vi "Main-Auto.vi"() -> ()   [LabVIEW 2019]
uses:
  <vilib>/Platform/TimedLoop/XDataNode/timing_clust.ctl
  <vilib>/Platform/TimedLoop/XDataNode/nitl_modes.ctl
  <vilib>/Platform/TimedLoop/XDataNode/wakeup.ctl
  <vilib>/myRIO/Instrument Drivers/Onboard IO/DIO/typedefs/DIO Reference.ctl
  <vilib>/myRIO/Common/Instrument Driver Framework/Utilities/typedefs/myRIO Generic Hardware Reference.ctl
  <vilib>/myRIO/Common/Instrument Driver Framework/Utilities/typedefs/Hardware Version Enum.ctl
  <vilib>/myRIO/Common/Instrument Driver Framework/Utilities/typedefs/myRIO v1.0 Reference.ctl
  <vilib>/myRIO/Common/Instrument Driver Framework/Utilities/typedefs/Generic FPGA Reference.ctl
  <vilib>/myRIO/Common/Instrument Driver Framework/myRIO v1.0/DIO/typedefs/DIO Channels List.ctl
  <vilib>/myRIO/Common/Instrument Driver Framework/myRIO v1.0/DIO/typedefs/DIO Channels Enum.ctl
  <vilib>/userDefined/High Color/nirio_resource_hc.ctl
  <vilib>/myRIO/Common/Instrument Driver Framework/Utilities/vis/Is FPGA Ref Available.vi
  <vilib>/myRIO/Common/Instrument Driver Framework/myRIO v1.0/DIO/vis/myRIO v1.1 Open DIO.vi
  <vilib>/myRIO/Instrument Drivers/Onboard IO/DIO/vis/Write.vi
  <vilib>/myRIO/Common/Instrument Driver Framework/Utilities/vis/Validate Channels.vi
  <vilib>/myRIO/Common/Instrument Driver Framework/myRIO v1.0/DIO/vis/myRIO v1.0 Reserve DIO.vi
  <vilib>/myRIO/Common/Instrument Driver Framework/myRIO v1.0/UART/vis/myRIO v1.0 Close UART.vi
  <vilib>/myRIO/Common/Instrument Driver Framework/myRIO v1.0/Resource Manager/vis/myRIO v1.0 Reserve Channel List.vi
  <vilib>/myRIO/Common/Instrument Driver Framework/myRIO v1.0/DIO/vis/myRIO v1.0 Build MUX Configuration DIO.vi
  <vilib>/myRIO/Common/Instrument Driver Framework/myRIO v1.0/Resource Manager/vis/myRIO v1.0 Reserve Channel.vi
  <vilib>/myRIO/Common/Instrument Driver Framework/myRIO v1.0/Resource Manager/vis/myRIO v1.0 Unreserve Channel.vi
  <vilib>/myRIO/Common/Instrument Driver Framework/myRIO v1.0/Resource Manager/vis/myRIO v1.0 Create Configuration List.vi
  <vilib>/myRIO/Common/Instrument Driver Framework/myRIO v1.0/Resource Manager/vis/myRIO v1.0 Build Mutex Name.vi
  Sub VI/Variable/Lock-PID.vi
  <vilib>/Utility/VariantDataType/GetNumericInfo.vi
  <vilib>/Utility/error.llb/Error Cluster From Error Code.vi
  <vilib>/myRIO/Common/Instrument Driver Framework/myRIO v1.0/myRIO v1.1 Open.vi
  <vilib>/myRIO/Common/Instrument Driver Framework/Utilities/vis/IO Manager.vi
  <vilib>/myRIO/Common/Instrument Driver Framework/Utilities/vis/Configuration Manager.vi
  <vilib>/myRIO/Common/Instrument Driver Framework/myRIO v1.0/Resource Manager/vis/myRIO v1.0 Configure IO.vi
  <vilib>/myRIO/Common/Instrument Driver Framework/myRIO v1.0/myRIO v1.0 Close.vi
  <vilib>/myRIO/Common/Instrument Driver Framework/myRIO v1.0/DIO/vis/myRIO v1.0 Write DIO.vi
  Sub VI/Variable/Go-Home.vi
  <vilib>/myRIO/Common/Instrument Driver Framework/Utilities/vis/FPGA Ref Manager.vi
  <vilib>/myRIO/Common/Instrument Driver Framework/myRIO v1.0/myRIO v1.0 Reset FPGA.vi
  <vilib>/myRIO/Common/Instrument Driver Framework/myRIO v1.0/IRQ/vis/myRIO v1.0 IRQ Info FGV.vi
  <vilib>/myRIO/Common/Instrument Driver Framework/myRIO v1.0/IRQ/vis/myRIO v1.0 Timer IRQ Info FGV.vi
  <vilib>/myRIO/Common/Instrument Driver Framework/myRIO v1.0/IRQ/vis/myRIO v1.0 ISR Agent.vi
  <vilib>/myRIO/Instrument Drivers/Utilities/vis/Reset Index.vi
  <vilib>/myRIO/Common/Instrument Driver Framework/myRIO v1.0/Resource Manager/vis/myRIO v1.0 Block Write Resource Manager.vi
  <vilib>/platform/TimedLoop/XDataNode/XDataNode.xnode
  <vilib>/myRIO/Express VI/Onboard Devices/LED/LED Express VI.xnode
  <vilib>/myRIO/Instrument Drivers/Onboard IO/DIO/vis/myRIO DIO Open.xnode
  <vilib>/myRIO/Instrument Drivers/Utilities/Utilities.lvlib
  <vilib>/Platform/TimedLoop/XDataNode/XDNodeRunTimeDep.lvlib
  <vilib>/myRIO/Instrument Drivers/Onboard IO/DIO/DIO.lvlib
panel:
  out "總辨識機率":i32[](graph)
  out "第二次辨識機率":i32[](graph)
  out "第一次辨識機率":i32[](graph)
  out "辨識機率":dbl[](array[slide]) scale=0.0..10.0
  out "總辨識結果":string[](array[string])
  out "輸出顏色-位置":T1(array[cluster])
  out "當前動作":enum16{"辨識", "夾球+回橋"}(ring)
  in  "Stop":bool
  out "Error Out":errorcluster
  in  "Error In":errorcluster
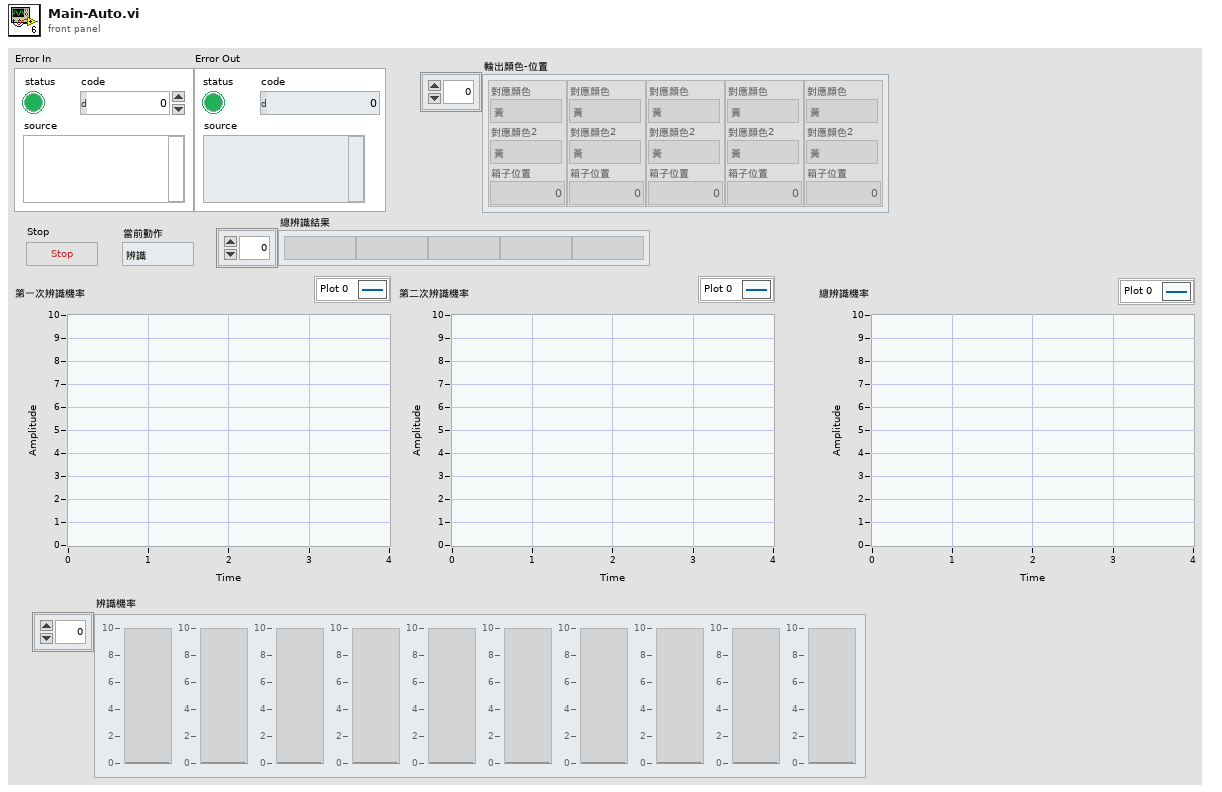
[diagram p1: front panel]
types:
  T1 = cluster{"對應顏色":enum16{"黃", "紅", "綠", "藍", "黑", "無"}, "對應顏色2":enum16{"黃", "紅", "綠", "藍", "黑", "無"}, "箱子位置":i32}[]
  T2 = enum16{"第一次夾球", "第二次夾球", "第三次夾球", "第四次夾球", "第五次夾球"}
  T3 = enum16{"第一次夾球", "第二次夾球", "第三次夾球", "第四次夾球", "第五次夾球"}[]
  T4 = typedef "I2C.lvlib/I2C Reference.ctl" = cluster{"myRIO Reference":T5, "I2C Channels Enum":T9, "I2C Configuration":T10}
  T5 = typedef "myRIO Generic Hardware Reference.ctl" = cluster{"myRIO Model":T6, "myRIO Hardware Reference":T7}
  T6 = typedef "Hardware Version Enum.ctl" = enum16{"Unknown", "myRIO-1900", "myRIO-1950", "roboRIO", "NI ELVIS RIO CM", "ELVIS III"}
  T7 = typedef "myRIO v1.0 Reference.ctl" = cluster{"Generic FPGA Reference":T8, "Allow multiple opens":bool}
  T8 = typedef "Generic FPGA Reference.ctl" = refnum<k20>
  T9 = typedef "I2C Channels Enum.ctl" = enum16{"Not Connected", "A/I2C", "B/I2C", "I2C/I2C"}
  T10 = typedef "I2C.lvlib/I2C Configuration.ctl" = cluster{"I2C Transfer Rate":T11}
  T11 = typedef "I2C.lvlib/I2C Transfer Rate.ctl" = enum16{"Standard mode (100 kbps)", "Fast mode (400 kbps)"}
  T12 = cluster{"Array":i32[], "Array":i32[], "Array":i32[]}
  T13 = typedef "XDNodeRunTimeDep.lvlib/timing_clust.ctl" = cluster{"Expected End [f-1]":u64, "Actual End [f-1]":u64, "Finished Late? [f-1]":bool, "Expected End [i-1]":u64, "Actual End [i-1]":u64, "Finished Late? [i-1]":bool, "Expected Start [i]":u64, "Actual Start [i]":u64, "Expected Start [f]":u64, "Actual Start [f]":u64, "Source Name":string, "Structure Name":string, "Period":i64, "Deadline":i64, "Offset":i64, "Start":i64, "Priority":i32, "Timeout":i32, "Mode":T14, "Wakeup Reason":T15, "Error":errorcluster, "Source Type":string, "Secondary Source Type":string, "Global End Time":u64, "Global Start Time":u64, "Frame Duration":u64, "Iteration Duration":u64, "Assigned CPU":i32, "I/O Scan Engine Mode":u32}
  T14 = typedef "XDNodeRunTimeDep.lvlib/nitl_modes.ctl" = enum32{"No Change", "Process missed periods, maintain original phase", "Discard missed periods, maintain original phase", "Process missed periods, ignore original phase", "Discard missed periods, ignore original phase"}
  T15 = typedef "XDNodeRunTimeDep.lvlib/wakeup.ctl" = enum32{"Normal", "Aborted", "Asynchronous wakeup", "Timing source error", "Timed loop error", "Timeout"}
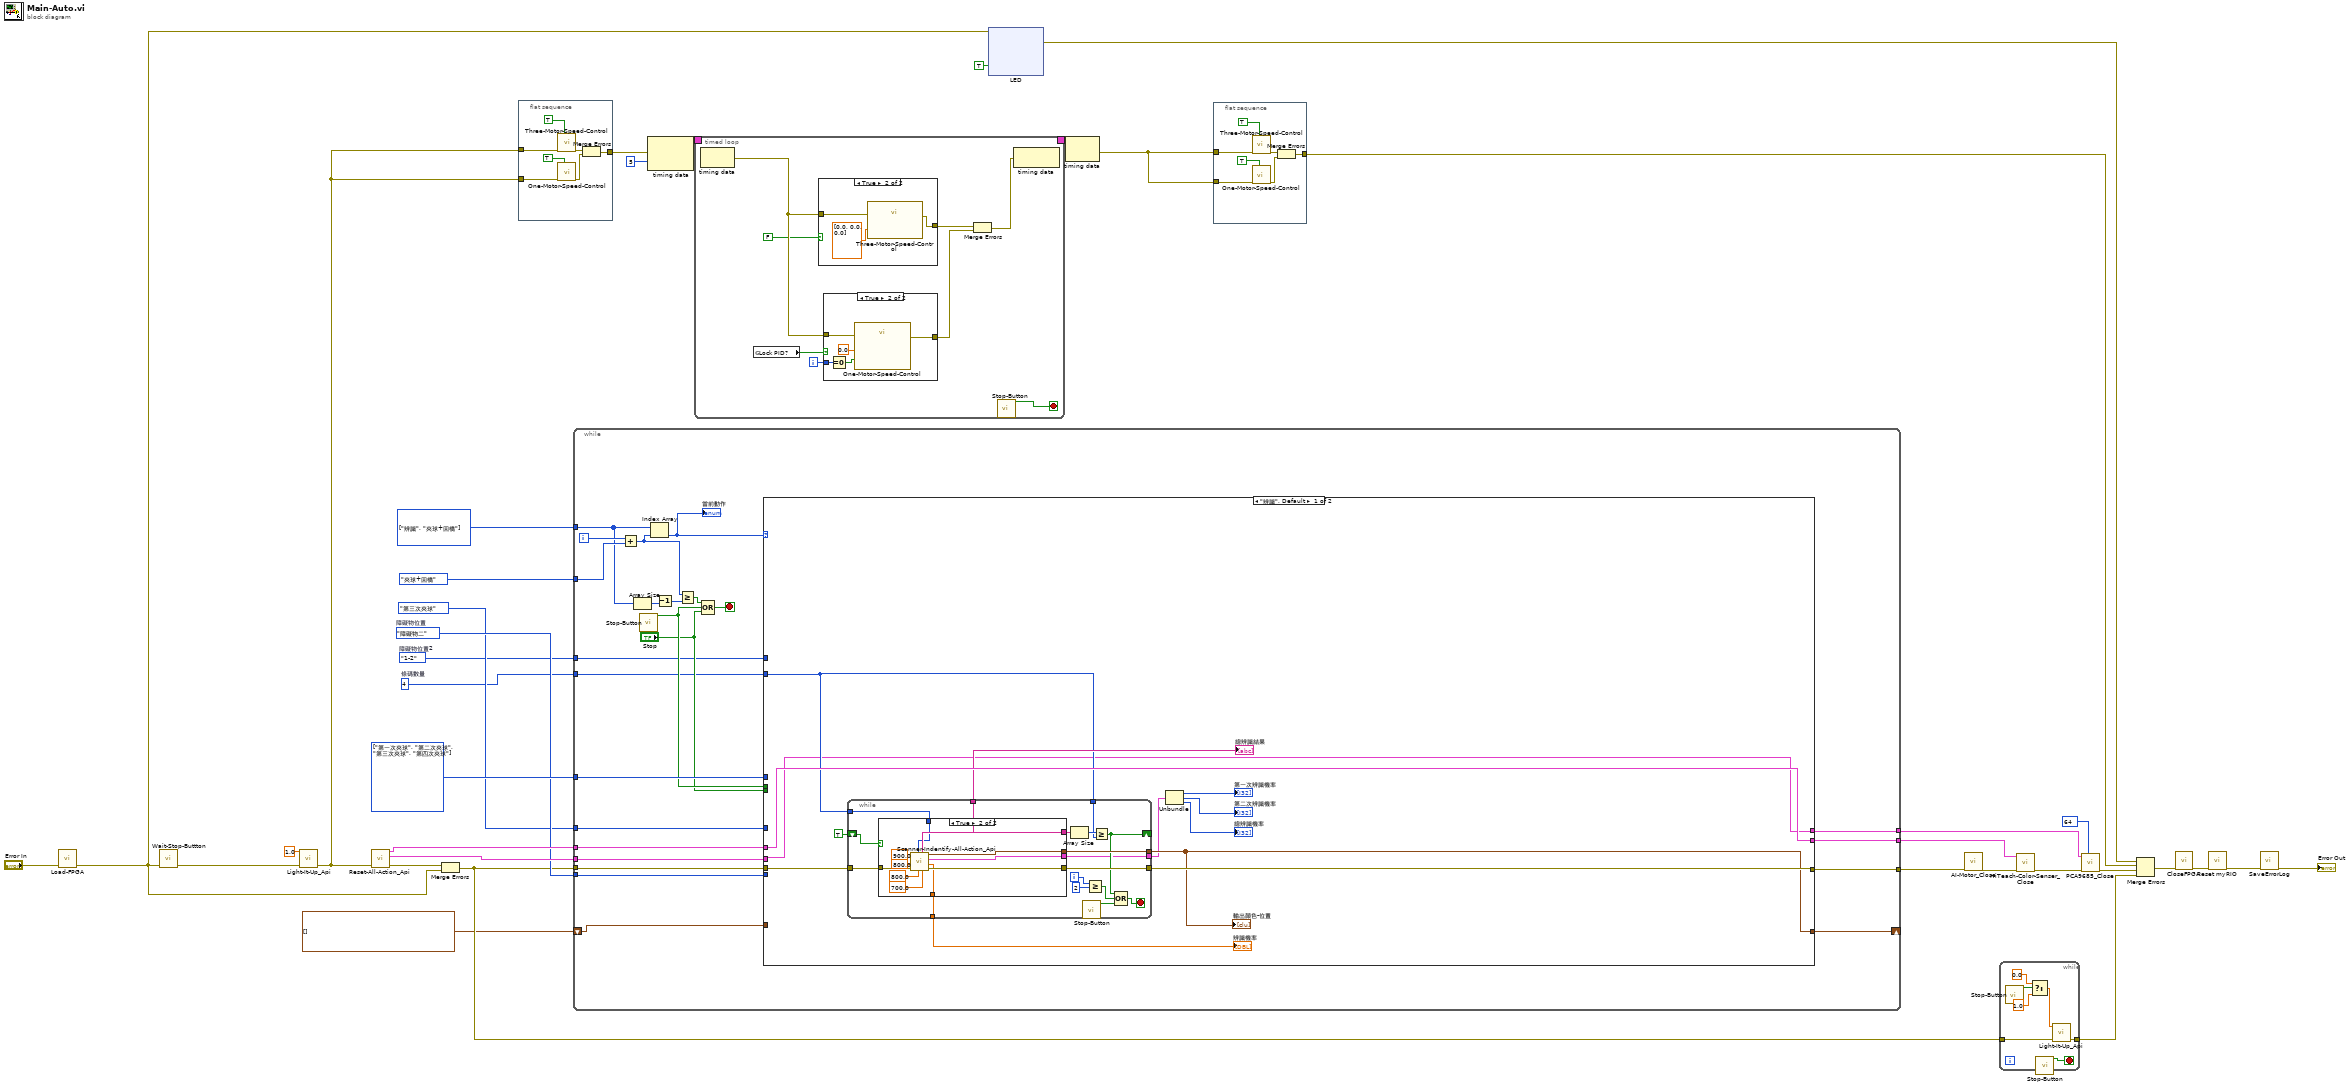
[diagram p0: block diagram]
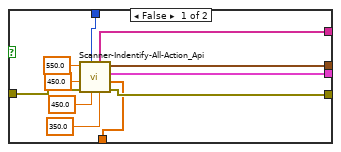
[diagram p2: hidden frame]
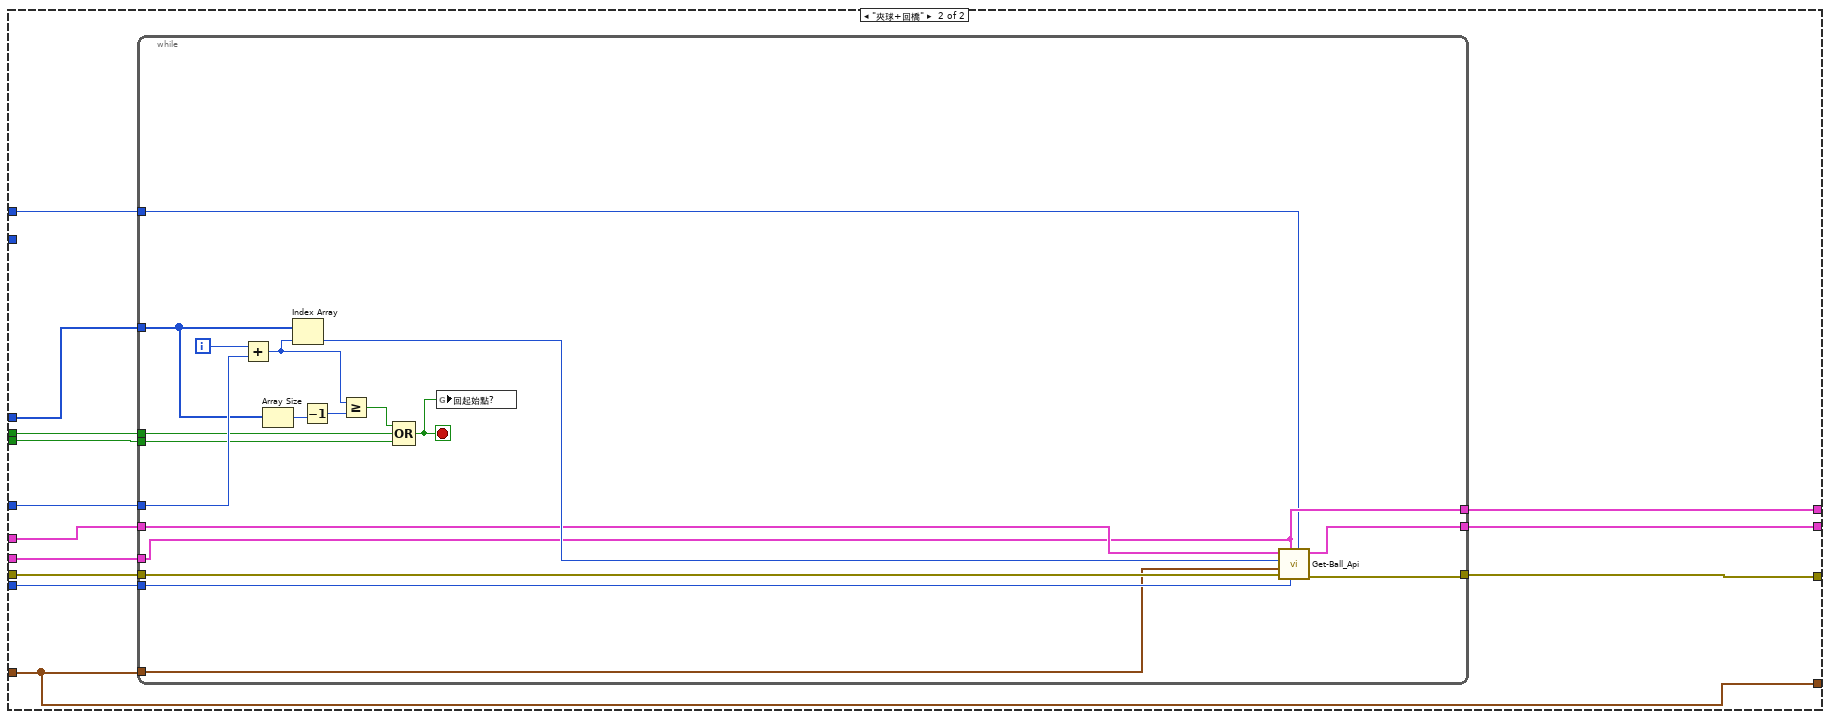
[diagram p3: hidden frame]
diagram:
  w3 = 4  # 條碼數量
  w5 = enum16{"1-1", "1-2", "2-1", "2-2"}."1-2"  # 障礙物位置2
  w19 = enum16{"障礙物一", "障礙物二"}."障礙物二"  # 障礙物位置
  w34 = T3 [enum."第一次夾球", enum."第二次夾球", enum."第三次夾球", enum."第四次夾球"] items=["第一次夾球", "第二次夾球", "第三次夾球", "第四次夾球", "第五次夾球"]
  w37 = enum16{"辨識", "夾球+回橋"}[] [enum."辨識", enum."夾球+回橋"] items=["辨識", "夾球+回橋"]
  n1 = call "Load-FPGA.vi"("Error In"="Error In") -> ("Error Out"=w7:errorcluster)  [unwired: 10 in]
  n2 = call "Wait-Stop-Buttton.vi"("Error In"=w7) -> ("Error Out"=w18:errorcluster)  [unwired: 10 in]
  n3 = call "Light-It-Up_Api.vi"("error in (no error)"=w18, "Duty Cycle"=1.0) -> ("error out"=w17:errorcluster)  [unwired: 9 in]
  n4 = call "Reset-All-Action_Api.vi"("Error In"=w17) -> ("Error Out"=w32:errorcluster, "I2C Ref Out"=w27:T4, "HiTechnicColorSensorV2 Ref Out"=w30:cluster{"I2C Ref Out":T4})  [unwired: 8 in]
  n5 = Merge Errors(w32, w7) -> (w13:errorcluster)
  n6 = flat-sequence {
    tunnel: w17 -> [w44]
    tunnel: w17 -> [w43]
    tunnel: [w40] -> w20
    frame #0 {
      n7 = call "Three-Motor-Speed-Control.vi"("Reset"=TRUE, "Error In"=w44) -> ("Error Out"=w42:errorcluster)  [unwired: 9 in]
      n8 = call "One-Motor-Speed-Control.vi"("Reset"=TRUE, "Error In"=w43) -> ("Error Out"=w41:errorcluster)  [unwired: 9 in]
      n9 = Merge Errors(w42, w41) -> (w40:errorcluster)
    }
  }
  n10 = while {
    tunnel: w37 -> [w58]
    tunnel: enum16{"辨識", "夾球+回橋"}."夾球+回橋" -> [w68]
    tunnel: w13 -> [w67]
    tunnel: [w66] -> w4
    tunnel: T2."第三次夾球" ("夾球開始位置") -> [w63]
    tunnel: w34 -> [w57]
    shift-right: [w54] -> _
    shift-left: T1 [] ("輸出顏色-位置") -> [w53]
    tunnel: w30 -> [w51]
    tunnel: [w50] -> w29
    tunnel: w27 -> [w47]
    tunnel: [w49] -> w28
    tunnel: w19 -> [w48]
    tunnel: w5 -> [w46]
    tunnel: w3 -> [w45]
    i -> [w64]
    stop <- w65 stop-if-true
    n11 = Add(x=w64, y=w68) -> (x+y=w61:i32)
    n12 = Array Size(array=w58) -> (size(s)=w60:i32)
    n13 = call "Stop-Button.vi"() -> ("顯示按下?"=w56:bool)  [unwired: 10 in, 1 out]
    n14 = Index Array(array=w58, index=w61) -> (element=w52:enum16{"辨識", "夾球+回橋"})
    "當前動作" <- w52
    n15 = Decrement(x=w60) -> (x-1=w59:i32)
    n16 = Greater Or Equal?(x=w61, y=w59) -> (x >= y?=w62:bool)
    n17 = Compound Arithmetic op=OR(w62, w56, "Stop") -> (w65:bool)
    n18 = case shown="\"辨識\", Default" w52 {
      tunnel: w67 -> [w80 w132]
      tunnel: [w79 w131] -> w66
      tunnel: w63 -> [_ w130]
      tunnel: w57 -> [_ w129]
      tunnel: w56 -> [_ w128]
      tunnel: "Stop" -> [_ w127]
      tunnel: [w78 w126] -> w54
      tunnel: w53 -> [_ w126]
      tunnel: w51 -> [w81 w125]
      tunnel: [w81 w124] -> w50
      tunnel: w47 -> [w69 w123]
      tunnel: [w69 w122] -> w49
      tunnel: w48 -> [_ w121]
      tunnel: w46 -> [_ w120]
      tunnel: w45 -> [w75 _]
      frame "辨識", Default {
        n19 = while {
          tunnel: w80 -> [w97]
          tunnel: [w94] -> w79
          tunnel: [w93] -> w78
          tunnel: [w88] -> w77
          shift-right: [w87] -> _
          shift-left: TRUE -> [w86]
          tunnel: w75 -> [w85]
          tunnel: w75 -> [w84]
          tunnel: [w83] -> w74
          tunnel: [w82] -> w70
          i -> [w92]
          stop <- w95 stop-if-true
          n20 = case shown="True" w86 {
            tunnel: w97 -> [w106 w119]
            tunnel: [w107 w118] -> w94
            tunnel: [w108 w117] -> w93
            tunnel: [w100 w116] -> w88
            tunnel: w85 -> [w101 w113]
            tunnel: [w99 w110] -> w83
            tunnel: [w98 w109] -> w82
            frame False {
              n21 = call "Scanner-Indentify-All-Action_Api.vi"("加速度 (回頭)"=350.0, "最高速 (回頭)"=450.0, "Barcode數量"=w101, "Error In"=w106, "加速度"=450.0, "最高速"=550.0) -> ("error out"=w107:errorcluster, 1:"辨識機率"=w98:dbl[], 2:"辨識機率"=w99:T12, "輸出顏色-位置"=w108:T1, "總辨識結果"=w100:string[])  [unwired: 1 in]
            }
            frame True {
              n22 = call "Scanner-Indentify-All-Action_Api.vi"("加速度 (回頭)"=700.0, "最高速 (回頭)"=800.0, "Barcode數量"=w113, "Error In"=w119, "加速度"=800.0, "最高速"=900.0) -> ("error out"=w118:errorcluster, 1:"辨識機率"=w109:dbl[], 2:"辨識機率"=w110:T12, "輸出顏色-位置"=w117:T1, "總辨識結果"=w116:string[])  [unwired: 1 in]
            }
          }
          n23 = Array Size(array=w88) -> (size(s)=w96:i32)
          n24 = call "Stop-Button.vi"() -> ("顯示按下?"=w89:bool)  [unwired: 10 in, 1 out]
          n25 = Greater Or Equal?(x=w92, y=2) -> (x >= y?=w90:bool)
          n26 = Greater Or Equal?(x=w96, y=w84) -> (x >= y?=w87:bool)
          n27 = Compound Arithmetic op=OR(w87, w90, w89) -> (w95:bool)
        }
        "輸出顏色-位置" <- w78
        "總辨識結果" <- w77
        "辨識機率" <- w70
        n28 = Unbundle(w74) -> ("Array"=→"第一次辨識機率":i32[], "Array"=→"第二次辨識機率":i32[], "Array"=→"總辨識機率":i32[])
      }
      frame "夾球+回橋" {
        n29 = while {
          tunnel: w130 -> [w145]
          tunnel: w129 -> [w144]
          tunnel: w128 -> [w143]
          tunnel: w127 -> [w142]
          tunnel: w126 -> [w134]
          tunnel: w125 -> [w140]
          tunnel: [w139] -> w124
          tunnel: w123 -> [w138]
          tunnel: w132 -> [w151]
          tunnel: [w133] -> w131
          tunnel: [w138] -> w122
          tunnel: w121 -> [w137]
          tunnel: w120 -> [w135]
          i -> [w146]
          stop <- w136 stop-if-true
          n30 = Add(x=w146, y=w145) -> (x+y=w150:i32)
          n31 = Array Size(array=w144) -> (size(s)=w149:i32)
          n32 = Index Array(array=w144, index=w150) -> (element=w141:T2)
          n33 = Decrement(x=w149) -> (x-1=w148:i32)
          n34 = Greater Or Equal?(x=w150, y=w148) -> (x >= y?=w147:bool)
          n35 = Compound Arithmetic op=OR(w147, w143, w142) -> (w136:bool)
          n36 = global write "Go-Home.vi" "回起始點?"(w136) -> ()
          n37 = call "Get-Ball_Api.vi"("障礙物位置2"=w135, "障礙物位置"=w137, "I2C Ref In"=w138, "Error In"=w151, "輸出顏色-位置"=w134, "夾球開始位置"=w141, "HiTechnicColorSensorV2 Ref"=w140) -> ("Error Out"=w133:errorcluster, "HiTechnicColorSensorV2 Ref Out"=w139:cluster{"I2C Ref Out":T4})  [unwired: 2 in, 1 out]
        }
      }
    }
  }
  n38 = node-c288(w20, i64 5 ("Period")) -> (w25:T13)
  n39 = timed-loop {
    timing: w25 -> [_]
    timing-out: [_] -> w24
    i -> [w152]
    stop <- w159 stop-if-true
    n40 = node-c288() -> (w158:errorcluster)  [unwired: 1 in]
    n41 = global read "Lock-PID.vi" "Lock PID?"() -> (w153:bool)
    n42 = case shown="True" FALSE {
      tunnel: w158 -> [w160 w161]
      tunnel: [w160 w162] -> w155
      frame False {
      }
      frame True {
        n43 = call "Three-Motor-Speed-Control.vi"("Error In"=w161, "速度(秒/度)"=dbl[] [0.0, 0.0, 0.0]) -> ("Error Out"=w162:errorcluster)  [unwired: 9 in]
      }
    }
    n44 = case shown="True" w153 {
      tunnel: w158 -> [w164 w168]
      tunnel: [w164 w167] -> w156
      tunnel: w152 -> [_ w166]
      frame False {
      }
      frame True {
        n45 = Equal To 0?(x=w166) -> (x = 0?=w165:bool)
        n46 = call "One-Motor-Speed-Control.vi"("Reset"=w165, "Error In"=w168, "速度(秒/度)"=0.0) -> ("Error Out"=w167:errorcluster)  [unwired: 8 in]
      }
    }
    n47 = Merge Errors(w155, w156) -> (w157:errorcluster)
    n48 = call "Stop-Button.vi"() -> ("顯示按下?"=w159:bool)  [unwired: 10 in, 1 out]
    n49 = node-c288(w157) -> ()  [unwired: 1 out]
  }
  n50 = xnode "LED"("LED1"=TRUE, "error in (no error)"=w7) -> ("error out"=w11:errorcluster)
  n51 = node-c288(w24) -> (w21:errorcluster)
  n52 = flat-sequence {
    tunnel: w21 -> [w181]
    tunnel: w21 -> [w180]
    tunnel: [w177] -> w12
    frame #0 {
      n53 = call "Three-Motor-Speed-Control.vi"("Reset"=TRUE, "Error In"=w181) -> ("Error Out"=w179:errorcluster)  [unwired: 9 in]
      n54 = call "One-Motor-Speed-Control.vi"("Reset"=TRUE, "Error In"=w180) -> ("Error Out"=w178:errorcluster)  [unwired: 9 in]
      n55 = Merge Errors(w179, w178) -> (w177:errorcluster)
    }
  }
  n56 = call "AI-Motor_Close.vi"("Error In"=w4) -> ("Error Out"=w26:errorcluster)  [unwired: 10 in]
  n57 = while {
    tunnel: w13 -> [w183]
    tunnel: [w188] -> w15
    stop <- w182 stop-if-true
    n58 = call "Stop-Button.vi"() -> ("顯示按下?"=w186:bool)  [unwired: 10 in, 1 out]
    n59 = Select(t=0.0, s=w186, f=1.0) -> (s? t:f=w187:dbl)
    n60 = call "Stop-Button.vi"() -> ("顯示按下?"=w182:bool)  [unwired: 10 in, 1 out]
    n61 = call "Light-It-Up_Api.vi"("error in (no error)"=w183, "Duty Cycle"=w187) -> ("error out"=w188:errorcluster)  [unwired: 9 in]
  }
  n62 = call "HiTeach-Color-Senser_Close.vi"("Error In"=w26, "HiTechnicColorSensorV2 Ref"=w29) -> ("Error Out"=w6:errorcluster)  [unwired: 9 in]
  n63 = call "PCA9685_Close.vi"("驅動板位址(0x40)"=u8 64, "Error In"=w6, "I2C Ref In"=w28) -> ("Error Out"=w22:errorcluster)  [unwired: 8 in]
  n64 = Merge Errors(w11, w12, w22, w15) -> (w14:errorcluster)
  n65 = call "CloseFPGA.vi"("Error In"=w14) -> ("Error Out"=w35:errorcluster)  [unwired: 10 in]
  n66 = call <vilib>:"Reset myRIO.vi"("error in (no error)"=w35) -> ("error out"=w2:errorcluster)  [unwired: 10 in]
  n67 = call "SaveErrorLog.vi"("Error In"=w2) -> ("error out"=→"Error Out":errorcluster)  [unwired: 10 in]
